vi "Configure Calib Linear (IO).vi"(0 "VISA resource name":refnum<visa-resource-name>, 5 "Channel (0001)":string="0001", 7 "Mode (0: Off)":u16(ring) items=["Off", "Apporoximation", "Bias"], 9 "Linearizer Input/Output":cluster{"Input":i32, "Output":i32}[](array[cluster]) {"Output" min=-999999 max=999999; "Input" min=-999999 max=999999}, 11 "error in (no error)":errorcluster) -> (4 "VISA resource name out":refnum<visa-resource-name>, 6 "Channel":string, 15 "error out":errorcluster)   [LabVIEW 2020, in "Yokogawa GX Series.lvlib"]
doc: "Sets the calibration correction(Linearizer Approximation and Linearizer Bias) for AI channels.\n\nCommand: SCalibIO"
uses:
  <instrlib>/Yokogawa GX Series/Yokogawa GX Series.lvlib
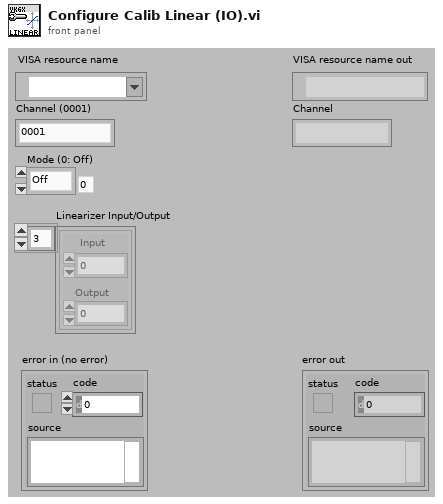
[diagram p1: front panel]
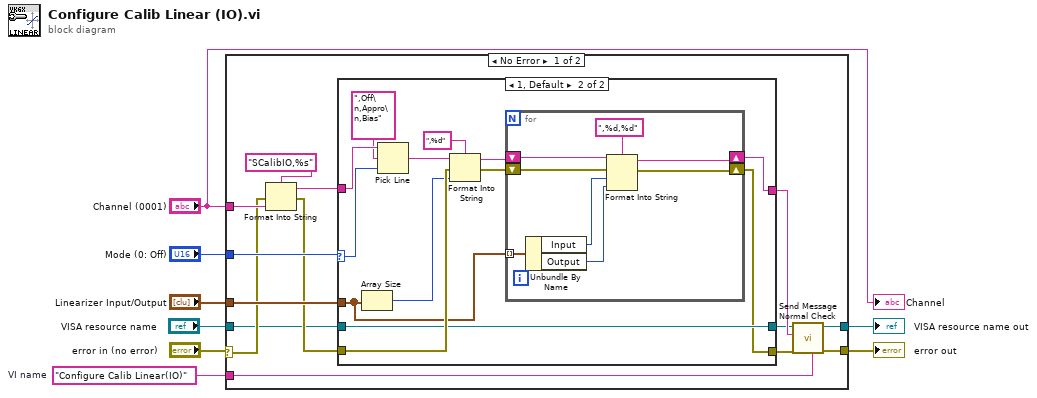
[diagram p0: block diagram]
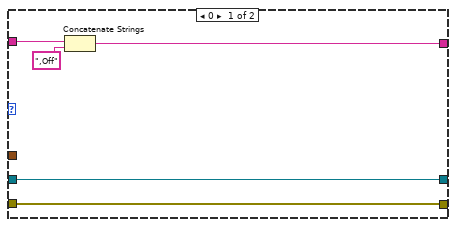
[diagram p2: hidden frame]
diagram:
  w8 = "Configure Calib Linear(IO)"  # VI name
  n1 = case shown="No Error" "error in (no error)" {
    selector: "error in (no error)" -> [w12 w49]
    tunnel: w8 -> [w22 _]
    tunnel: [w21 w50] -> w7
    tunnel: [w20 w49] -> w6
    tunnel: "VISA resource name" -> [w11 w50]
    tunnel: "Mode (0: Off)" -> [w18 _]
    tunnel: "Linearizer Input/Output" -> [w16 _]
    tunnel: "Channel (0001)" -> [w14 _]
    frame No Error {
      n2 = Format Into String(format string="SCalibIO,%s", error in=w12, w14) -> (resulting string=w17:string, error out=w15:errorcluster)  [unwired: 1 in]
      n3 = case shown="1, Default" w18 {
        selector: w18 -> [_ w40]
        tunnel: w17 -> [w27 w39]
        tunnel: [w25 w31] -> w13
        tunnel: w16 -> [_ w33]
        tunnel: w15 -> [w23 w35]
        tunnel: w11 -> [w24 w30]
        tunnel: [w24 w30] -> w10
        tunnel: [w23 w29] -> w9
        frame 0 {
          n4 = Concatenate Strings(w27, ",Off") -> (w25:string)
        }
        frame 1, Default {
          n5 = Array Size(array=w33) -> (size(s)=w28:i32)
          n6 = Pick Line(string ("")=w39, multi-line string=",Off\n,Appro\n,Bias", line index=w40) -> (output string=w36:string)
          n7 = Format Into String(format string=",%d", initial string=w36, error in=w35, w28) -> (resulting string=w34:string, error out=w32:errorcluster)
          n8 = for {
            tunnel: w33 -> [w46] mode=indexing
            shift-right: [w42] -> w31
            shift-left: w34 -> [w48]
            shift-right: [w43] -> w29
            shift-left: w32 -> [w47]
            n9 = Unbundle By Name(w46) -> ("Input"=w45:i32, "Output"=w44:i32)
            n10 = Format Into String(format string=",%d,%d", initial string=w48, error in=w47, w45, w44) -> (resulting string=w42:string, error out=w43:errorcluster)
          }
        }
      }
      n11 = call <instrlib>:"Send Message Normal Check.vi"("Source (\"\")"=w22, "error in (no error)"=w9, "Send Message (\"\")"=w13, "VISA resource name"=w10) -> ("error out"=w20:errorcluster, "VISA resource name out"=w21:refnum<visa-resource-name>)  [unwired: 2 in, 4 out]
    }
    frame Error {
    }
  }
  "error out" <- w6
  "VISA resource name out" <- w7
  "Channel" <- "Channel (0001)"
